vi "ADS1256 Stop.vi"(10 "Channel":i8, 11 "DevHandle":i32) -> (3 "function return":i32)   [LabVIEW 2010, in "usb2ads1256.lvlib"]
doc: "int WINAPI ADS1256_Stop(int DevHandle,char Channel);"
uses:
  usb2ads1256.lvlib
  USB2XXX.dll
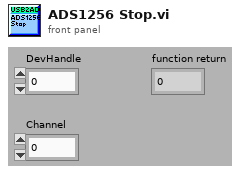
[diagram p1: front panel]
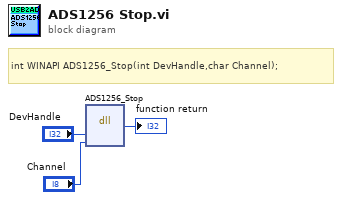
[diagram p0: block diagram]
diagram:
  # "int WINAPI ADS1256_Stop(int DevHandle,char Channel);"
  n1 = dll-call lib="G:/OtherWork/USB2XXX_Example/trunk/Labview/PublicFiles/usb2ads1256/USB2XXX.*" fn="ADS1256_Stop"("DevHandle"="DevHandle", "Channel"="Channel") -> (→"function return":i32)  [unwired: 5 in, 2 out]
